vi "VITester_Provider_Startup.vi"(8 "error in (no error)":errorcluster, 11 "Project Refnum":refnum<vi>) -> (0 "error out":errorcluster)   [LabVIEW 2009]
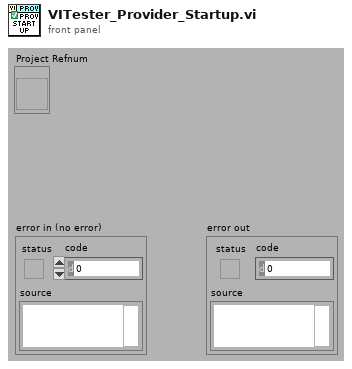
[diagram p1: front panel]
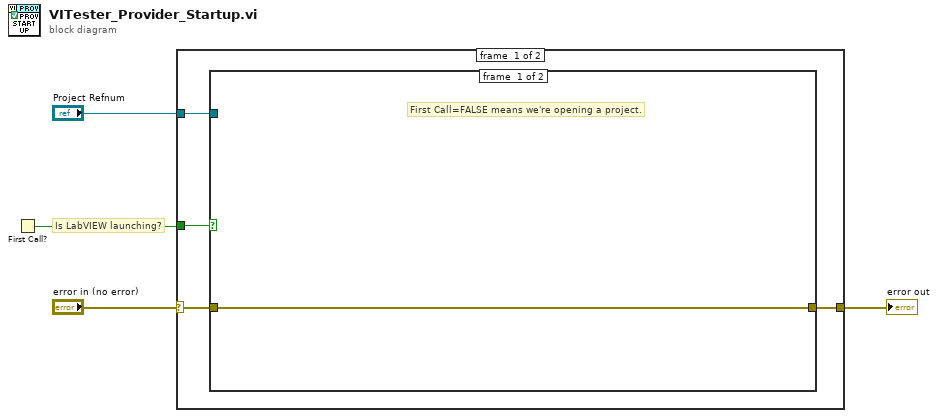
[diagram p0: block diagram]
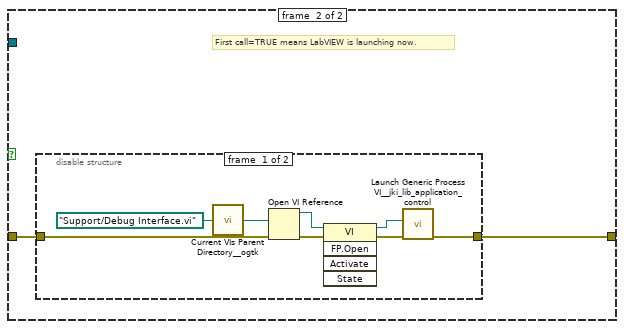
[diagram p2: hidden frame]
diagram:
  # "Is LabVIEW launching?"
  n1 = First Call?() -> (First Call?: T/F=w2:bool)
  n2 = case shown="No Error" "error in (no error)" {
    selector: "error in (no error)" -> [w8 w21]
    tunnel: [w7 w21] -> w3
    tunnel: w2 -> [w6 _]
    tunnel: "Project Refnum" -> [w5 _]
    frame #0 {
      n3 = case shown="True" w6 {
        tunnel: w8 -> [w9 w11]
        tunnel: [w9 w10] -> w7
        tunnel: w5 -> [_ _]
        frame #0 {
          # "First Call=FALSE means we're opening a project."
        }
        frame #1 {
          # "First call=TRUE means LabVIEW is launching now."
          n4 = disable-structure shown="Enabled" {
            disable-tunnel: w11 -> [w17 w20]
            disable-tunnel: [w16 w20] -> w10
            frame #0 {
              n5 = call <userlib>:"Current VIs Parent Directory__ogtk.vi"("Relative path (.)"=path "Support/Debug Interface.vi") -> ("Parent Directory (+ Relative)"=w19:path)  [unwired: 4 in]
              n6 = Open VI Reference(vi path=w19, error in (no error)=w17) -> (vi reference=w12:refnum<vi>, error out=w14:errorcluster)  [unwired: 4 in]
              n7 = invoke class="VI" method="FP.Open"(reference=w12, error in=w14) -> (reference out=w13:refnum<vi>, error out=w15:errorcluster)  [unwired: 3 in, 3 out]
              n8 = call <vilib>:"Launch Generic Process VI__jki_lib_application_control.vi"("error out"=w15, "Process VI RefNum"=w13) -> ("error"=w16:errorcluster)  [unwired: 7 in, 2 out]
            }
            frame #1 {
            }
          }
        }
      }
    }
    frame #1 {
    }
  }
  "error out" <- w3
